vi "Get SMO Port.vi"(8 "error in (no error)":errorcluster, 11 "Inst.Attocube-3DRInstrument in":refnum<class "Inst.Attocube-3DR.lvclass">) -> (0 "error out":errorcluster, 2 "Port":u16, 3 "Inst.Attocube-3DRInstrument out":refnum<class "Inst.Attocube-3DR.lvclass">)   [LabVIEW 2019, in "Inst.Attocube-3DR.lvclass"]
uses:
  Inst.Attocube-3DR.lvclass
  <userlib>/LevyLab/Instrument Framework/Instrument Types/VSource/Instrument.VSource.lvclass
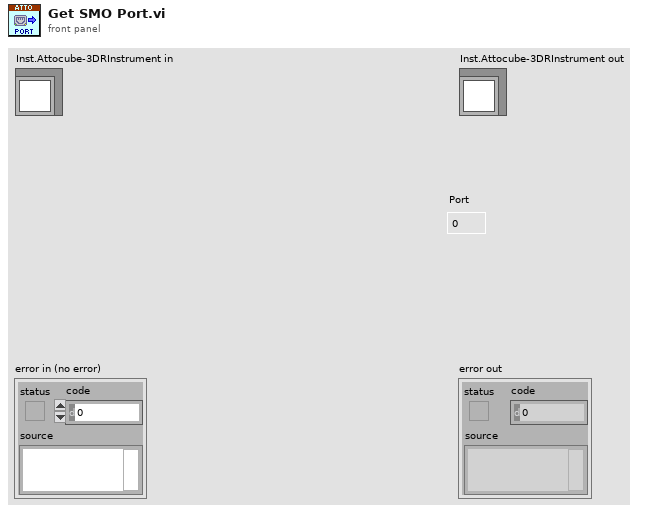
[diagram p1: front panel]
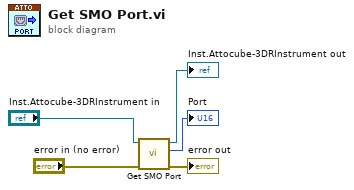
[diagram p0: block diagram]
diagram:
  n1 = call-parent "Get SMO Port.vi"("error in (no error)"="error in (no error)", "Instrument in"="Inst.Attocube-3DRInstrument in") -> ("error out"=→"error out":errorcluster, "Port"=→"Port":u16, "Instrument out"=→"Inst.Attocube-3DRInstrument out":refnum<class "Inst.Attocube-3DR.lvclass">)  [unwired: 7 in]
